vi "JAUS In from Q Out.vi"   [LabVIEW 2009]
uses:
  <vilib>/Platform/TimedLoop/XDataNode/XDataNode.xnode
  <vilib>/Platform/TimedLoop/XDataNode/loadlvalarms.vi
  <vilib>/Platform/TimedLoop/XDataNode/timing_clust.ctl
  <vilib>/Platform/TimedLoop/XDataNode/nitl_modes.ctl
  <vilib>/Platform/TimedLoop/XDataNode/wakeup.ctl
  cRIO/Functional Global Variables/Actions for FG's.ctl
  Support Files/VelocityState.ctl
  Support Files/TimeRec.ctl
  Support Files/LocalPose.ctl
  <vilib>/Platform/TimedLoop/XDataNode/XDNodeRunTimeDep.lvlib
types:
  T1 = typedef "XDNodeRunTimeDep.lvlib/timing_clust.ctl" = cluster{"Expected End [f-1]":u64, "Actual End [f-1]":u64, "Finished Late? [f-1]":bool, "Expected End [i-1]":u64, "Actual End [i-1]":u64, "Finished Late? [i-1]":bool, "Expected Start [i]":u64, "Actual Start [i]":u64, "Expected Start [f]":u64, "Actual Start [f]":u64, "Source Name":string, "Structure Name":string, "Period":i64, "Deadline":i64, "Offset":i64, "Start":i64, "Priority":i32, "Timeout":i32, "Mode":T2, "Wakeup Reason":T3, "Error":errorcluster, "Source Type":string, "Secondary Source Type":string, "Global End Time":u64, "Global Start Time":u64, "Frame Duration":u64, "Iteration Duration":u64, "Assigned CPU":i32, "I/O Scan Engine Mode":u32}
  T2 = typedef "XDNodeRunTimeDep.lvlib/nitl_modes.ctl" = enum32{"No Change", "Process missed periods, maintain original phase", "Discard missed periods, maintain original phase", "Process missed periods, ignore original phase", "Discard missed periods, ignore original phase"}
  T3 = typedef "XDNodeRunTimeDep.lvlib/wakeup.ctl" = enum32{"Normal", "Aborted", "Asynchronous wakeup", "Timing source error", "Timed loop error", "Timeout"}
  T4 = typedef "Actions for FG's.ctl" = enum16{"Read", "Write"}
  T5 = typedef "VelocityState.ctl" = cluster{"Velocity X":dbl, "Velocity Y":dbl, "Velocity Z":dbl, "Velocity RMS":dbl, "Roll Rate":dbl, "Pitch Rate":dbl, "Yaw Rate":dbl, "Rate RMS":dbl, "TimeRec":T6}
  T6 = typedef "TimeRec.ctl" = cluster{"Milliseconds":u32, "Seconds":u32, "Minutes":u32, "Hours":u32, "Day":u32}
  T7 = typedef "LocalPose.ctl" = cluster{" X":dbl, " Y":dbl, " Z":dbl, "Position RMS":dbl, "Roll":dbl, "Pitch":dbl, "Yaw":dbl, "Attitude RMS":dbl, "TimeRec":T6}
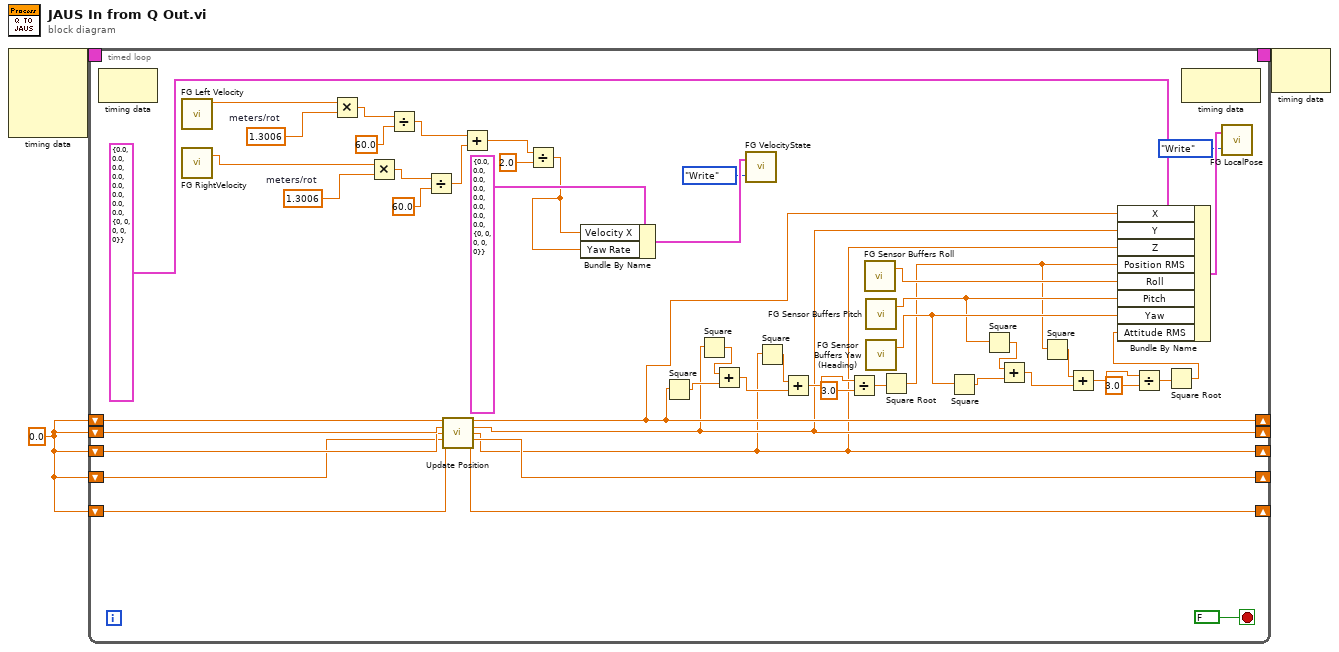
[diagram p0: block diagram]
diagram:
  w1 = 0.0 ("Last Position X")
  n1 = node-c288() -> (w3:T1)  [unwired: 4 in]
  n2 = timed-loop {
    timing: w3 -> [_]
    timing-out: [_] -> w2
    shift-right: [w21] -> _
    shift-left: w1 -> [w38]
    shift-right: [w20] -> _
    shift-left: w1 -> [w37]
    shift-right: [w19] -> _
    shift-left: w1 -> [w36]
    shift-right: [w34] -> _
    shift-left: w1 -> [w35]
    shift-right: [w32] -> _
    shift-left: w1 -> [w33]
    stop <- FALSE stop-if-true
    w48 = 1.3006  # meters/rot
    w51 = 1.3006  # meters/rot
    n3 = node-c288() -> ()  [unwired: 1 in, 1 out]
    n4 = call "FG Left Velocity.vi"() -> ("Left Velocity Out (RPM)"=w52:dbl)  [unwired: 3 in]
    n5 = call "FG RightVelocity.vi"() -> ("Right Velocity Out (RPM)"=w45:dbl)  [unwired: 3 in]
    n6 = Multiply(x=w52, y=w51) -> (x*y=w50:dbl)
    n7 = Multiply(x=w45, y=w48) -> (x*y=w47:dbl)
    n8 = Divide(x=w50, y=60.0) -> (x/y=w43:dbl)
    n9 = Divide(x=w47, y=60.0) -> (x/y=w42:dbl)
    n10 = call "Update Position.vi"("Last Position X"=w38, "Last Postion Y"=w37, "Last Postion Z"=w36, "Last Left Dist"=w35, "Last Right Dist"=w33) -> ("New X"=w21:dbl, "New Y"=w20:dbl, "New Z"=w19:dbl, "Left Dist Travelled Out (cm)"=w34:dbl, "Right Dist Travelled Out (cm)"=w32:dbl)  [unwired: 6 in]
    n11 = Add(x=w43, y=w42) -> (x+y=w41:dbl)
    n12 = Divide(x=w41, y=2.0) -> (x/y=w6:dbl)
    n13 = Bundle By Name(cluster=T5 {"Velocity X"=0.0, "Velocity Y"=0.0, "Velocity Z"=0.0, "Velocity RMS"=0.0, "Roll Rate"=0.0, "Pitch Rate"=0.0, "Yaw Rate"=0.0, "Rate RMS"=0.0, "TimeRec"={"Milliseconds"=0, "Seconds"=0, "Minutes"=0, "Hours"=0, "Day"=0}} ("VelocityState in"), "Velocity X"=w6, "Yaw Rate"=w6) -> (w40:T5)
    n14 = Square(x=w21) -> (x^2=w26:dbl)
    n15 = Square(x=w20) -> (x^2=w25:dbl)
    n16 = Add(x=w25, y=w26) -> (x+y=w24:dbl)
    n17 = call "FG VelocityState.vi"("FG Action (Read)"=Actions_for_FG's."Write", "VelocityState in"=w40) -> ()  [unwired: 1 out]
    n18 = Square(x=w19) -> (x^2=w23:dbl)
    n19 = Add(x=w23, y=w24) -> (x+y=w22:dbl)
    n20 = Divide(x=w22, y=3.0) -> (x/y=w27:dbl)
    n21 = call "FG Sensor Buffers Roll.vi"() -> ("Roll Buffer out"=w18:dbl)  [unwired: 3 in]
    n22 = call "FG Sensor Buffers Pitch.vi"() -> ("Pitch Buffer out"=w10:dbl)  [unwired: 3 in]
    n23 = call "FG Sensor Buffers Yaw (Heading).vi"() -> ("Yaw Buffer Out"=w11:dbl)  [unwired: 3 in]
    n24 = Square Root(x=w27) -> (sqrt(x)=w9:dbl)
    n25 = Square(x=w11) -> (x^2=w15:dbl)
    n26 = Square(x=w10) -> (x^2=w8:dbl)
    n27 = Add(x=w8, y=w15) -> (x+y=w14:dbl)
    n28 = Square(x=w9) -> (x^2=w13:dbl)
    n29 = Add(x=w13, y=w14) -> (x+y=w12:dbl)
    n30 = Divide(x=w12, y=3.0) -> (x/y=w16:dbl)
    n31 = Square Root(x=w16) -> (sqrt(x)=w7:dbl)
    n32 = Bundle By Name(cluster=T7 {" X"=0.0, " Y"=0.0, " Z"=0.0, "Position RMS"=0.0, "Roll"=0.0, "Pitch"=0.0, "Yaw"=0.0, "Attitude RMS"=0.0, "TimeRec"={"Milliseconds"=0, "Seconds"=0, "Minutes"=0, "Hours"=0, "Day"=0}} ("LocalPose in"), "X"=w21, "Y"=w20, "Z"=w19, "Position RMS"=w9, "Roll"=w18, "Pitch"=w10, "Yaw"=w11, "Attitude RMS"=w7) -> (w29:T7)
    n33 = node-c288() -> ()  [unwired: 1 in, 1 out]
    n34 = call "FG LocalPose.vi"("FG Action (Read)"=Actions_for_FG's."Write", "LocalPose in"=w29) -> ()  [unwired: 1 out]
  }
  n35 = node-c288(w2) -> ()  [unwired: 1 out]
